vi "Get CCD_Config.vi"(8 "error in (no error)":errorcluster, 11 "Interface in":refnum<class "Interface.lvclass">) -> (0 "error out":errorcluster, 2 "output cluster":T1={"ACQUISITION_MODE"=1, "TRIGGER_MODE"=0, "READ_MODE"=4, "PREAMP"=0, "READOUT_RATE"=0, "VERTICAL_SHIFT_SPEED"=3, "EM_MODE"=0, "EM_GAIN"=2, "SHUTTER_MODE"=2, "SHUTTER_TTL"=0, "SHUTTER_OPENING_TIME"=50, "SHUTTER_CLOSING_TIME"=50, "VBIN"=1, "HBIN"=1, "INITIAL_LINE"=1, "INITIAL_COLUMN"=1, "FINAL_LINE"=1024, "FINAL_COLUMN"=1024, "FRAME_TRANSFER"=FALSE, "VERTICAL_CLOCK_VOLTAGE"=0, "AD_CHANNEL"=0} {"VERTICAL_CLOCK_VOLTAGE" items=["Normal", "+1", "+2", "+3", "+4"]; "SHUTTER_TTL" items=["TTL Low", "TTl High"]; "SHUTTER_MODE" items=["Fully Auto", "OPEN", "CLOSED"]; "EM_MODE" items=["Electron Multiplying", "Conventional"]; "VERTICAL_SHIFT_SPEED" items=["0.6", "1.13", "2.2", "4.33"]; "READOUT_RATE" items=["1 MHz", "10 MHz", "20 MHz", "30 MHz"]; "PREAMP" items=["Gain 1", "Gain 2"]; "READ_MODE" items=["Full Vertical Binning", "Multi-Track", "Random-track", "Single-Track", "Image"]; "TRIGGER_MODE" items=["Internal", "External", "N/A", "N/A", "N/A", "N/A", "External Start"]; "ACQUISITION_MODE" items=["N/A", "Single", "Accumulate", "Kinetic", "Fast Kinetic"]}, 3 "Interface out":refnum<class "Interface.lvclass">)   [LabVIEW 2018, in "Interface.lvclass"]
uses:
  Interface.lvclass
  Interface.lvclass/Interface.ctl
panel:
  out "EXPTIME":dbl
  out "#FRAMES":u32
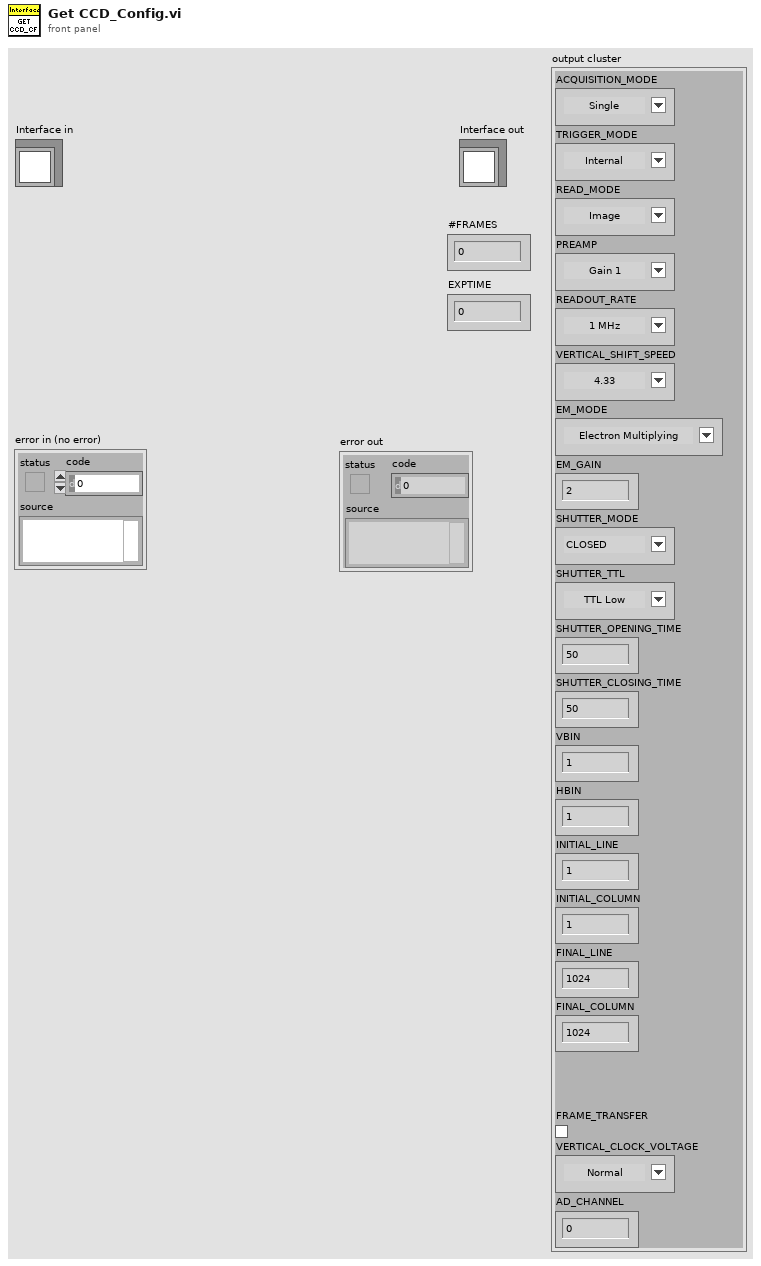
[diagram p1: front panel]
types:
  T1 = cluster{"ACQUISITION_MODE":u8, "TRIGGER_MODE":u8, "READ_MODE":u8, "PREAMP":u8, "READOUT_RATE":u8, "VERTICAL_SHIFT_SPEED":u8, "EM_MODE":u8, "EM_GAIN":u16, "SHUTTER_MODE":u8, "SHUTTER_TTL":u8, "SHUTTER_OPENING_TIME":u16, "SHUTTER_CLOSING_TIME":u16, "VBIN":u16, "HBIN":u16, "INITIAL_LINE":u16, "INITIAL_COLUMN":u16, "FINAL_LINE":u16, "FINAL_COLUMN":u16, "FRAME_TRANSFER":bool, "VERTICAL_CLOCK_VOLTAGE":u8, "AD_CHANNEL":u32}
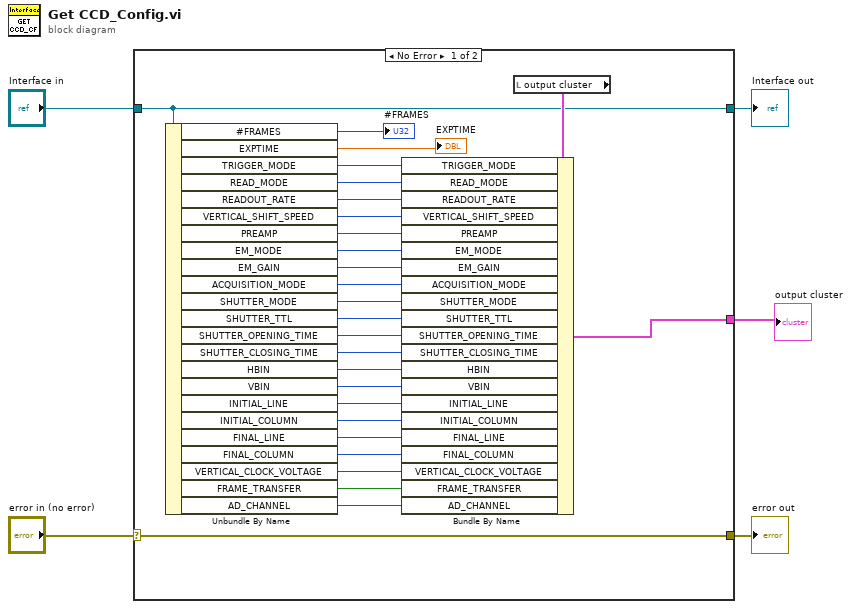
[diagram p0: block diagram]
diagram:
  n1 = case shown="No Error" "error in (no error)" {
    selector: "error in (no error)" -> [w32 w34]
    tunnel: [w32 w34] -> w4
    tunnel: [w8 w33] -> w2
    tunnel: "Interface in" -> [w8 w33]
    tunnel: [w9 _] -> w1
    frame No Error {
      n2 = Unbundle By Name(w8) -> ("#FRAMES"=→"#FRAMES":u32, "EXPTIME"=→"EXPTIME":dbl, "TRIGGER_MODE"=w31:u8, "READ_MODE"=w30:u8, "READOUT_RATE"=w29:u8, "VERTICAL_SHIFT_SPEED"=w28:u8, "PREAMP"=w27:u8, "EM_MODE"=w26:u8, "EM_GAIN"=w25:u16, "ACQUISITION_MODE"=w24:u8, "SHUTTER_MODE"=w23:u8, "SHUTTER_TTL"=w22:u8, "SHUTTER_OPENING_TIME"=w21:i32, "SHUTTER_CLOSING_TIME"=w20:i32, "HBIN"=w19:u16, "VBIN"=w18:u16, "INITIAL_LINE"=w17:u16, "INITIAL_COLUMN"=w16:u16, "FINAL_LINE"=w15:u16, "FINAL_COLUMN"=w14:u16, "VERTICAL_CLOCK_VOLTAGE"=w13:u8, "FRAME_TRANSFER"=w12:bool, "AD_CHANNEL"=w11:u32)
      n3 = local read "output cluster"() -> (w10:T1)
      n4 = Bundle By Name(cluster=w10, "TRIGGER_MODE"=w31, "READ_MODE"=w30, "READOUT_RATE"=w29, "VERTICAL_SHIFT_SPEED"=w28, "PREAMP"=w27, "EM_MODE"=w26, "EM_GAIN"=w25, "ACQUISITION_MODE"=w24, "SHUTTER_MODE"=w23, "SHUTTER_TTL"=w22, "SHUTTER_OPENING_TIME"=w21, "SHUTTER_CLOSING_TIME"=w20, "HBIN"=w19, "VBIN"=w18, "INITIAL_LINE"=w17, "INITIAL_COLUMN"=w16, "FINAL_LINE"=w15, "FINAL_COLUMN"=w14, "VERTICAL_CLOCK_VOLTAGE"=w13, "FRAME_TRANSFER"=w12, "AD_CHANNEL"=w11) -> (w9:T1)
    }
    frame Error {
    }
  }
  "error out" <- w4
  "Interface out" <- w2
  "output cluster" <- w1
